vi "Test Classes.vi"() -> ()   [LabVIEW 2009]
uses:
  LV-BME Interface/ChnlSettings.ctl
  LV-BME Interface/BME_DG_TriggerSettings.ctl
  LV-BME Interface/ClockSource.ctl
  DG Classes/BME_DG_System/BME_DG_System.lvclass
  DG Classes/BME_DG_Base/BME_DG_Base.lvclass
  DG Classes/BME_DG_Chnl/BME_DG_Chnl.lvclass
panel:
  in  "SetDelay":bool=TRUE
  in  "UpdateChnl 2":bool=TRUE
  in  "ChnlParameter":T2 {"ChnParam2write"."Delay (µs)" min=0.0 max=100000000.0 format="%.5f"}
  out "CountsRemains":i32
  in  "Acknowledge Interrupts":bool=TRUE
  out "TriggerCounters":i32[](array[numeric])
  out "Interrupts":u32[](array[numeric]) format="%b"
  in  "ClockSource Master":T3=1 items=["Internal Oscillator"=1, "External Trigger"=2, "Trigger & Oscillator"=3, "MasterSlave Bus"=4]
  in  "Trigger Settings Slaves":T4={"InputTerminated?"=FALSE, "InternalClockPeriode(µs)"=1000000.0, "TriggerLevel"=1.25, "PresetValue"=0, "DivideBy"=1, "Clock Source"=1, "Gate Divider"=1, "PositiveGate?"=TRUE, "InternalTrigger?"=FALSE, "InternalArm?"=FALSE, "SWTrigger?"=FALSE, "RisingEdge?"=FALSE, "StopOnPreset?"=FALSE, "ResetWhenDone?"=TRUE, "TriggerEnabled?"=TRUE} {"Gate Divider" min=1 max=1000000; "Clock Source" items=["Internal Oscillator"=1, "External Trigger"=2, "Trigger & Oscillator"=3]}
  in  "Trigger Settings Master":T4={"InputTerminated?"=FALSE, "InternalClockPeriode(µs)"=1000000.0, "TriggerLevel"=1.25, "PresetValue"=0, "DivideBy"=1, "Clock Source"=1, "Gate Divider"=1, "PositiveGate?"=TRUE, "InternalTrigger?"=TRUE, "InternalArm?"=FALSE, "SWTrigger?"=FALSE, "RisingEdge?"=FALSE, "StopOnPreset?"=FALSE, "ResetWhenDone?"=TRUE, "TriggerEnabled?"=TRUE} {"Gate Divider" min=1 max=1000000; "Clock Source" items=["Internal Oscillator"=1, "External Trigger"=2, "Trigger & Oscillator"=3]}
  out "RemainingTriggers":T5(array[cluster])=[[{"Time Stamp"=timestamp(3416308194.6875 s since 1904-01-01), "Numeric"=-64}, {"Time Stamp"=timestamp(3416308194.6875 s since 1904-01-01), "Numeric"=4}, {"Time Stamp"=timestamp(3416308194.6875 s since 1904-01-01), "Numeric"=-64}, {"Time Stamp"=timestamp(3416308194.6875 s since 1904-01-01), "Numeric"=-64}], [{"Time Stamp"=timestamp(3416308194.6875 s since 1904-01-01), "Numeric"=-64}, {"Time Stamp"=timestamp(3416308194.6875 s since 1904-01-01), "Numeric"=-64}, {"Time Stamp"=timestamp(3416308194.6875 s since 1904-01-01), "Numeric"=-64}, {"Time Stamp"=timestamp(3416308194.6875 s since 1904-01-01), "Numeric"=-64}], [{"Time Stamp"=timestamp(3416308194.6875 s since 1904-01-01), "Numeric"=-64}, {"Time Stamp"=timestamp(3416308194.6875 s since 1904-01-01), "Numeric"=-64}, {"Time Stamp"=timestamp(3416308194.6875 s since 1904-01-01), "Numeric"=-64}, {"Time Stamp"=timestamp(3416308194.6875 s since 1904-01-01), "Numeric"=-64}]] {"Time Stamp" format="%<%I:%M:%S%3u %p>T"}
  in  "stop 2":bool=TRUE
  in  "ReadStatus":bool=TRUE
  in  "Activate":bool
  in  "UpdateChnl":bool=TRUE
  in  "TriggerModulo":u32=4
  out "Modulo Settings":u32[](array[numeric])
  out "Chnls":T1[](array[typedef])=[{" Delay (µs)"=0.0, "On? (false)"=TRUE, "PositiveVoltage?(true)"=TRUE, "50OhmTerminated? "=TRUE, "25OhmOutput?"=FALSE}, {" Delay (µs)"=0.0, "On? (false)"=TRUE, "PositiveVoltage?(true)"=TRUE, "50OhmTerminated? "=TRUE, "25OhmOutput?"=FALSE}, {" Delay (µs)"=0.0, "On? (false)"=TRUE, "PositiveVoltage?(true)"=TRUE, "50OhmTerminated? "=TRUE, "25OhmOutput?"=FALSE}] {"Delay (µs)" min=0.0 max=100000000.0 format="%.5f"}
  in  "Trigger Base":T4={"InputTerminated?"=FALSE, "InternalClockPeriode(µs)"=1000000.0, "TriggerLevel"=1.25, "PresetValue"=0, "DivideBy"=1, "Clock Source"=1, "Gate Divider"=1, "PositiveGate?"=TRUE, "InternalTrigger?"=FALSE, "InternalArm?"=FALSE, "SWTrigger?"=FALSE, "RisingEdge?"=FALSE, "StopOnPreset?"=FALSE, "ResetWhenDone?"=TRUE, "TriggerEnabled?"=TRUE} {"Gate Divider" min=1 max=1000000; "Clock Source" items=["Internal Oscillator"=1, "External Trigger"=2, "Trigger & Oscillator"=3]}
  in  "Selected Chnl":u16(ring) items=["Slave 1_ChnlT0", "Slave 1_ChnlA", "Slave 1_ChnlB"]
  in  "Selected Card":u16(ring)=1 items=["Master", "Slave 1", "Slave 2", "Slave 3"]
  in  "STOP":bool=TRUE
  in  "ChnParam2write":T1={" Delay (µs)"=0.0, "On? (false)"=TRUE, "PositiveVoltage?(true)"=TRUE, "50OhmTerminated? "=TRUE, "25OhmOutput?"=FALSE} {"Delay (µs)" min=0.0 max=100000000.0 format="%.5f"}
  # "INIT Values"
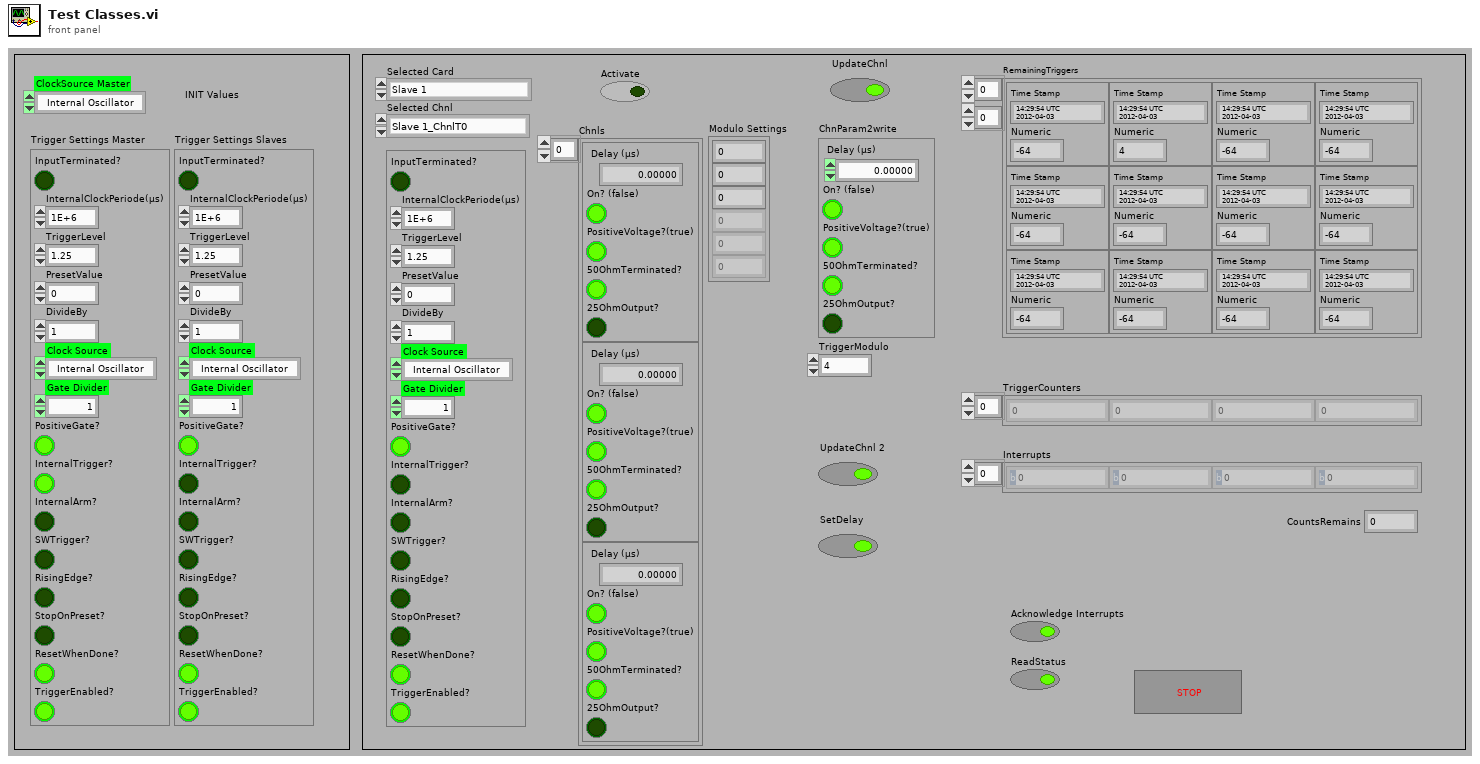
[diagram p1: front panel]
types:
  T1 = typedef "ChnlSettings.ctl" = cluster{" Delay (µs)":dbl, "On? (false)":bool, "PositiveVoltage?(true)":bool, "50OhmTerminated? ":bool, "25OhmOutput?":bool}
  T2 = cluster{"ChnlName":string, "ChnParam2write":T1, "TriggerModulo":u32}
  T3 = typedef "ClockSource.ctl" = i32
  T4 = typedef "BME_DG_TriggerSettings.ctl" = cluster{"InputTerminated?":bool, "InternalClockPeriode(µs)":dbl, "TriggerLevel":dbl, "PresetValue":i32, "DivideBy":i32, "Clock Source":u32, "Gate Divider":i32, "PositiveGate?":bool, "InternalTrigger?":bool, "InternalArm?":bool, "SWTrigger?":bool, "RisingEdge?":bool, "StopOnPreset?":bool, "ResetWhenDone?":bool, "TriggerEnabled?":bool}
  T5 = cluster{"Time Stamp":timestamp, "Numeric":i32}[][]
  T6 = enum8{"Enabled", "Disabled", "Disabled and Grayed Out"}
  T7 = cluster{"ChnlName":string, "ChnParam2write":T1, "TriggerModulo":u32}[]
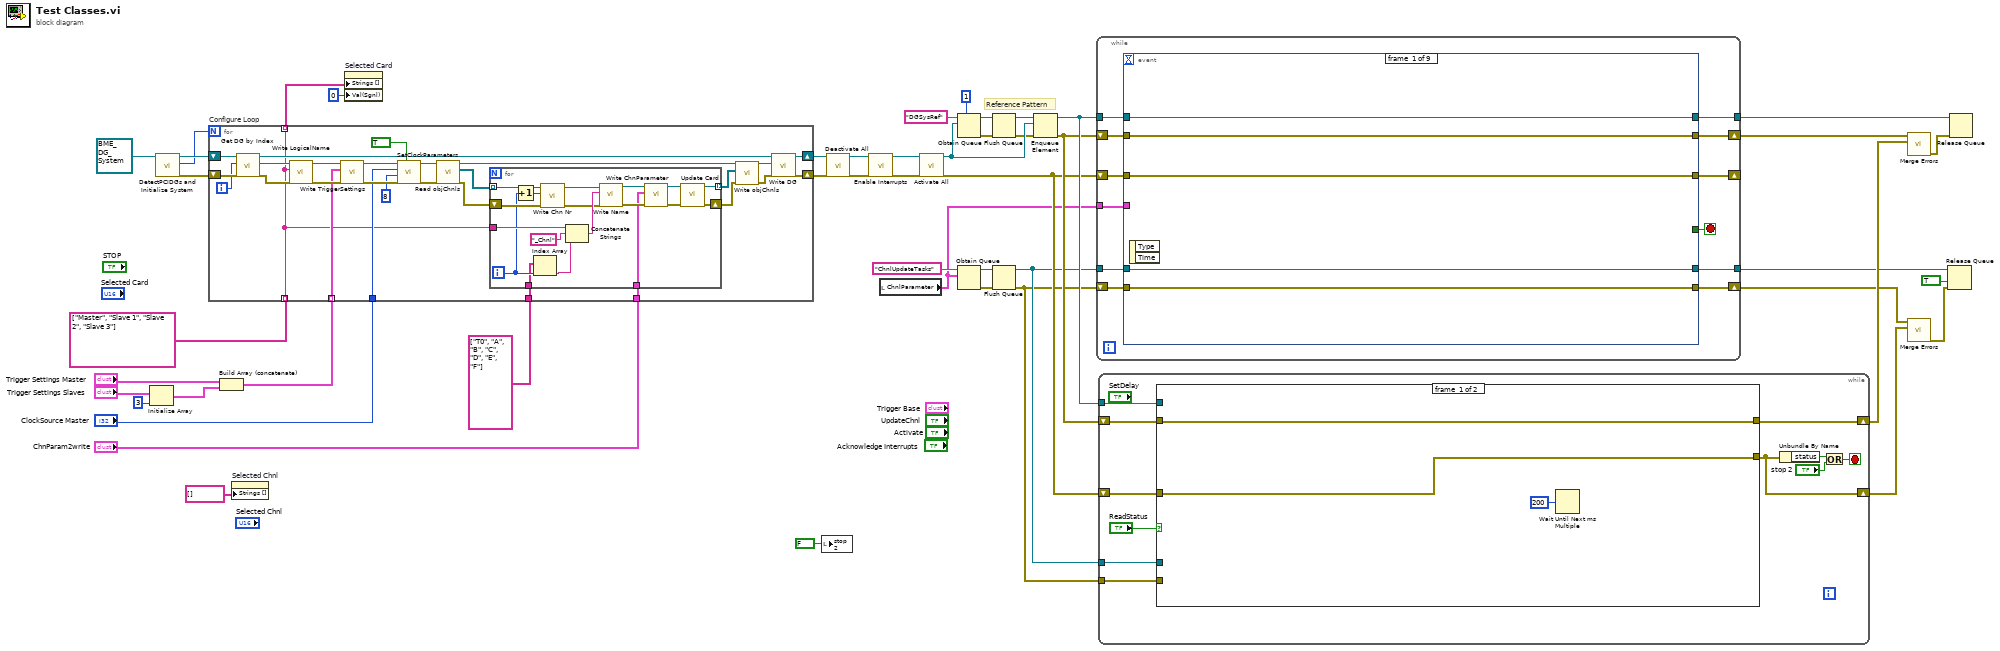
[diagram p0: block diagram]
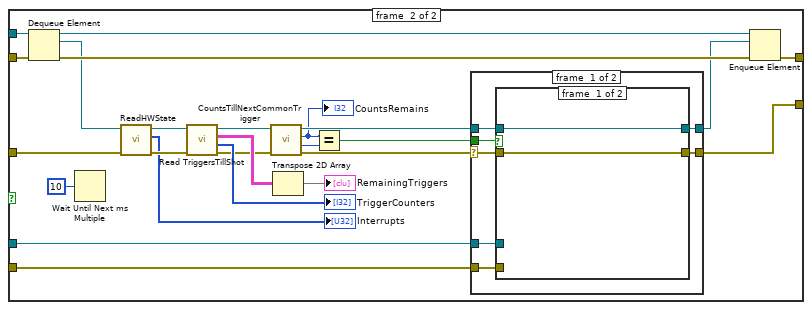
[diagram p2: hidden frame]
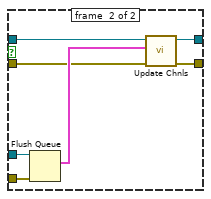
[diagram p3: hidden frame]
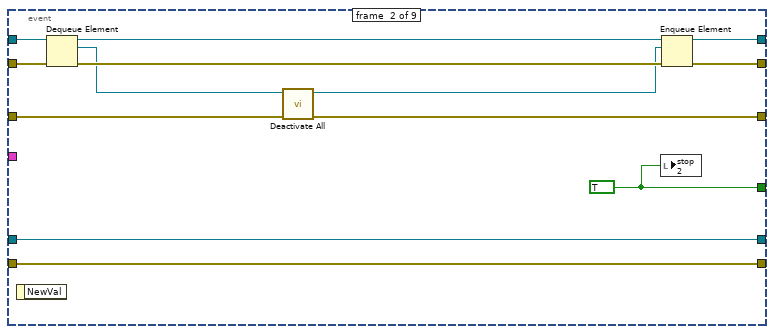
[diagram p5: hidden frame]
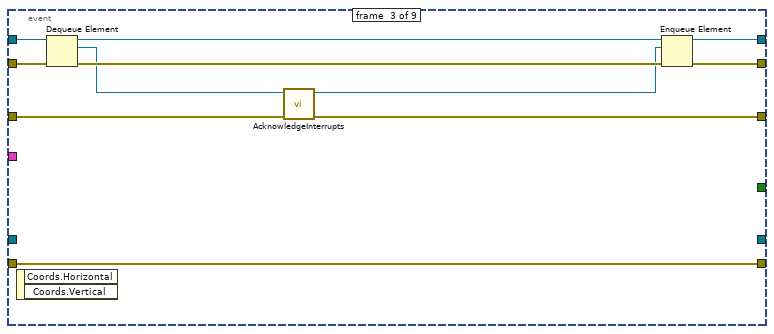
[diagram p6: hidden frame]
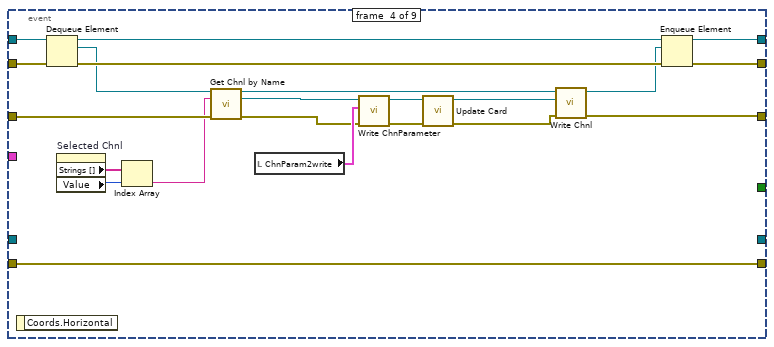
[diagram p7: hidden frame]
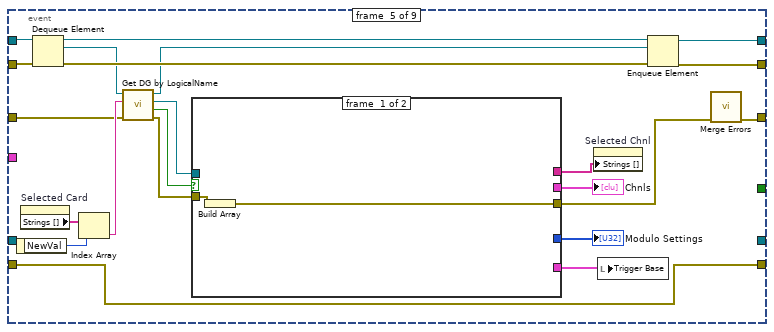
[diagram p8: hidden frame]
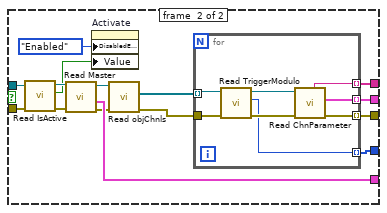
[diagram p9: hidden frame]
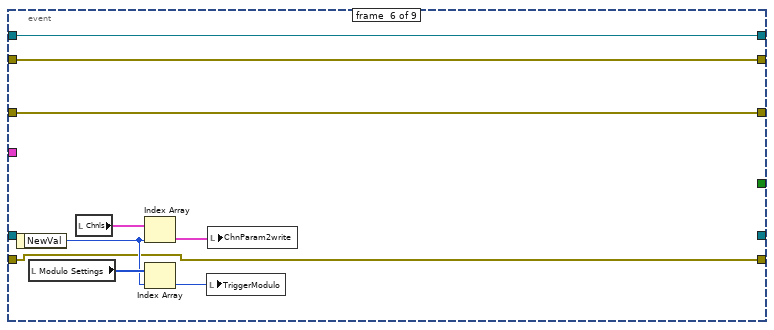
[diagram p10: hidden frame]
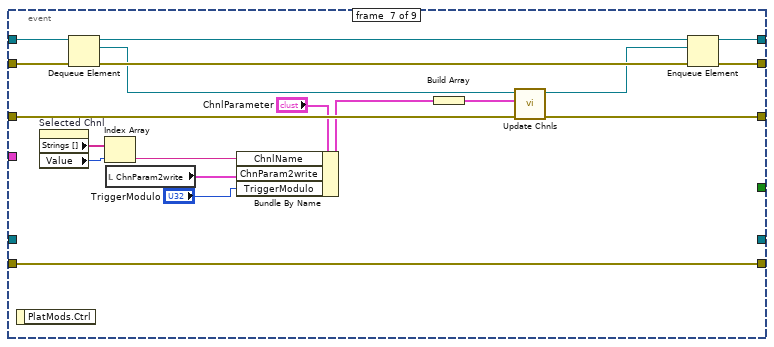
[diagram p11: hidden frame]
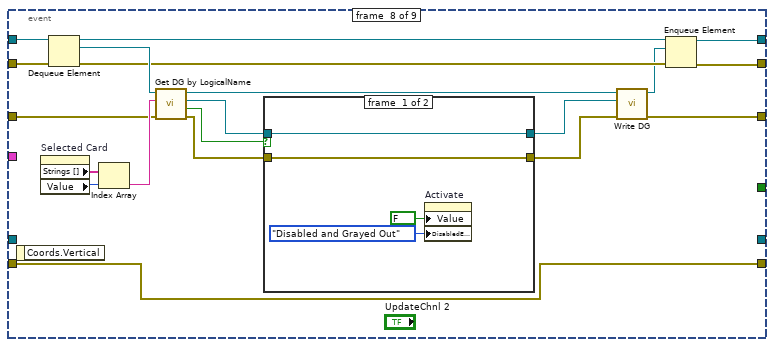
[diagram p12: hidden frame]
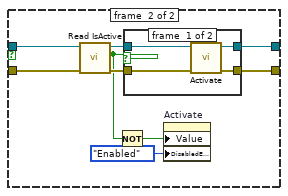
[diagram p13: hidden frame]
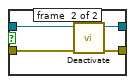
[diagram p14: hidden frame]
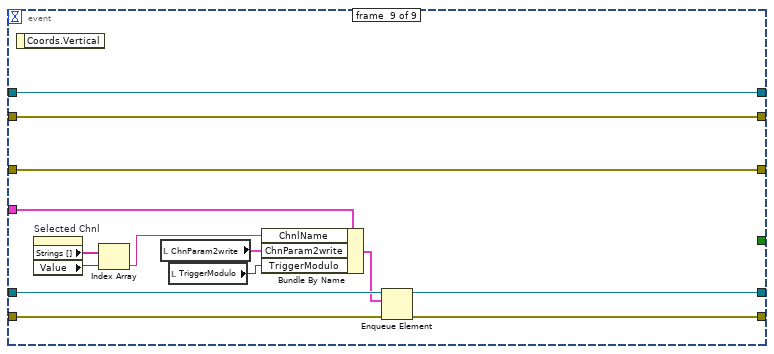
[diagram p15: hidden frame]
diagram:
  # "Reference Pattern"
  n1 = Initialize Array("Trigger Settings Slaves", 3 ("dimension size")) -> (w18:T4[])
  n2 = call "DetectPCIDGs and Initialize System.vi"("BME_DG_System in"=refnum<class "BME_DG_System.lvclass"> refnum ("BME_DG_System.lvclass")) -> ("error out"=w46:errorcluster, "NumberOfCards"=w45:i32, "BME_DG_System out"=w47:refnum<class "BME_DG_System.lvclass">)  [unwired: 8 in]
  n3 = Build Array (concatenate)("Trigger Settings Master", w18) -> (w21:T4[])
  n4 = for "Configure Loop" {
    N: w45 -> [_]
    shift-right: [w62] -> w39
    shift-left: w47 -> [w76]
    tunnel: string[] ["Master", "Slave 1", "Slave 2", "Slave 3"] -> [w49] mode=indexing
    tunnel: w21 -> [w67] mode=indexing
    tunnel: "ClockSource Master" -> [w64]
    shift-right: [w61] -> w38
    shift-left: w46 -> [w75]
    tunnel: "ChnParam2write" -> [w56]
    tunnel: string[] ["T0", "A", "B", "C", "D", "E", "F"] -> [w50]
    tunnel: [w49] -> w41 mode=indexing
    i -> [w74]
    n5 = call "Get DG by Index.vi"("error in (no error)"=w75, "index"=w74, "BME_DG_System in"=w76) -> ("error out"=w70:errorcluster, "BME_DG_Base.lvclass"=w73:refnum<class "BME_DG_Base.lvclass">, "BME_DG_System out"=w63:refnum<class "BME_DG_System.lvclass">)  [unwired: 6 in]
    n6 = call "Write LogicalName.vi"("error in (no error)"=w70, "LogicalName"=w49, "BME_DG_Base in"=w73) -> ("error out"=w69:errorcluster, "BME_DG_Base out"=w72:refnum<class "BME_DG_Base.lvclass">)  [unwired: 7 in]
    n7 = call-dynamic "Write TriggerSettings.vi"("error in (no error)"=w69, "Trigger Settings"=w67, "BME_DG_Base in"=w72) -> ("error out"=w68:errorcluster, "BME_DG_Base out"=w71:refnum<class "BME_DG_Base.lvclass">)  [unwired: 7 in]
    n8 = call-dynamic "SetClockParameters.vi"("ClockEnable"=TRUE, "error in (no error)"=w68, "DivideBy"=u32 8, "ClockSource"=w64, "BME_DG_Base in"=w71) -> ("error out"=w59:errorcluster, "BME_DG_Base out"=w60:refnum<class "BME_DG_Base.lvclass">)  [unwired: 5 in]
    n9 = call-dynamic "Read objChnls.vi"("error in (no error)"=w59, "BME_DG_Base in"=w60) -> ("error out"=w57:errorcluster, "objChnls"=w58:refnum<class "BME_DG_Chnl.lvclass">[], "BME_DG_Base out"=w54:refnum<class "BME_DG_Base.lvclass">)  [unwired: 6 in, 1 out]
    n10 = for {
      tunnel: w58 -> [w88] mode=indexing
      shift-right: [w77] -> w52
      shift-left: w57 -> [w86]
      tunnel: w49 -> [w93]
      tunnel: w56 -> [w89]
      tunnel: [w79] -> w55 mode=indexing
      tunnel: w50 -> [w82]
      i -> [w83]
      n11 = Increment(x=w83) -> (x+1=w84:i32)
      n12 = Index Array(array=w82, index=w83) -> (element=w81:string)
      n13 = call-dynamic "Write Chn Nr.vi"("error in (no error)"=w86, "Chn Nr"=w84, "BME_DG_Chnl in"=w88) -> ("error out"=w85:errorcluster, "BME_DG_Chnl out"=w87:refnum<class "BME_DG_Chnl.lvclass">)  [unwired: 7 in]
      n14 = Concatenate Strings(w93, "_Chnl" ("string"), w81) -> (w91:string)
      n15 = call-dynamic "Write Name.vi"("error in (no error)"=w85, "Name"=w91, "BME_DG_Chnl in"=w87) -> ("error out"=w90:errorcluster, "BME_DG_Chnl out"=w94:refnum<class "BME_DG_Chnl.lvclass">)  [unwired: 7 in]
      n16 = call-dynamic "Write ChnParameter.vi"("error in (no error)"=w90, "ChnParemater"=w89, "BME_DG_Chnl in"=w94) -> ("error out"=w78:errorcluster, "BME_DG_Chnl out"=w80:refnum<class "BME_DG_Chnl.lvclass">)  [unwired: 7 in]
      n17 = call-dynamic "Update Card.vi"("error in (no error)"=w78, "BME_DG_Chnl in"=w80) -> ("error out"=w77:errorcluster, "BME_DG_Chnl out"=w79:refnum<class "BME_DG_Chnl.lvclass">)  [unwired: 8 in]
    }
    n18 = call-dynamic "Write objChnls.vi"("error in (no error)"=w52, "objChnls"=w55, "BME_DG_Base in"=w54) -> ("error out"=w51:errorcluster, "BME_DG_Base out"=w53:refnum<class "BME_DG_Base.lvclass">)  [unwired: 7 in]
    n19 = call "Write DG.vi"("error in (no error)"=w51, "BME_DG_Base"=w53, "BME_DG_System in"=w63) -> ("error out"=w61:errorcluster, "BME_DG_System out"=w62:refnum<class "BME_DG_System.lvclass">)  [unwired: 7 in]
  }
  n20 = property on="Selected Chnl" class="Ring (strict)"("Strings []"=string[] []) -> ()  [unwired: 2 in, 2 out]
  n21 = property on="Selected Card" class="Ring (strict)"("Strings []"=w41, "Val(Sgnl)"=u16 0 ("Value (Signaling)")) -> ()  [unwired: 2 in, 2 out]
  n22 = local write "stop 2"(FALSE ("stop 2")) -> ()
  n23 = call "Deactivate All.vi"("error in (no error)"=w38, "BME_DG_System in"=w39) -> ("error out"=w12:errorcluster, "BME_DG_System out"=w15:refnum<class "BME_DG_System.lvclass">)  [unwired: 8 in]
  n24 = call "Enable Interrupts.vi"("error in (no error)"=w12, "BME_DG_System in"=w15) -> ("error out"=w13:errorcluster, "BME_DG_System out"=w14:refnum<class "BME_DG_System.lvclass">)  [unwired: 8 in]
  n25 = local read "ChnlParameter"() -> (w8:T2)
  n26 = call "Activate All.vi"("error in (no error)"=w13, "BME_DG_System in"=w14) -> ("error out"=w28:errorcluster, "BME_DG_System out"=w35:refnum<class "BME_DG_System.lvclass">)  [unwired: 8 in]
  n27 = Obtain Queue(max queue size (-1, unlimited)=1, name (unnamed)="DGSysRef", element data type=w35) -> (queue out=w26:refnum<queue>, error out=w24:errorcluster)  [unwired: 2 in, 1 out]
  n28 = Obtain Queue(name (unnamed)="ChnlUpdateTasks", element data type=w8) -> (queue out=w9:refnum<queue>, error out=w10:errorcluster)  [unwired: 3 in, 1 out]
  n29 = Flush Queue(queue=w26, error in (no error)=w24) -> (queue out=w25:refnum<queue>, error out=w23:errorcluster)  [unwired: 1 out]
  n30 = Flush Queue(queue=w9, error in (no error)=w10) -> (queue out=w5:refnum<queue>, error out=w4:errorcluster)  [unwired: 1 out]
  n31 = Enqueue Element(queue=w25, element=w35, error in (no error)=w23) -> (queue out=w34:refnum<queue>, error out=w33:errorcluster)  [unwired: 1 in, 1 out]
  n32 = while {
    shift-right: [w102] -> _
    shift-left: w28 -> [w104]
    shift-right: [w100] -> w30
    shift-left: w33 -> [w101]
    tunnel: w34 -> [w105]
    tunnel: [w103] -> w32
    tunnel: w5 -> [w99]
    tunnel: w8 -> [w98]
    tunnel: [w96] -> w7
    shift-right: [w95] -> w3
    shift-left: w4 -> [w97]
    stop <- w106 stop-if-true
    n33 = event shown="[3] \"SetDelay\": Mouse Down" {
      selector: _ -> [_ _ _ _ _ _ _ _ _]
      dyn-events: _ -> [_ _ _ _ _ _ _ _ _]
      timeout: _ -> [_ _ _ _ _ _ _ _ _]
      tunnel: [_ w114 _ _ _ _ _ _ _] -> w106
      tunnel: w105 -> [w111 w121 w134 w156 w167 w213 w230 w241 w287]
      tunnel: w104 -> [w110 w124 w126 w147 w176 w212 w222 w249 w286]
      tunnel: [w111 w117 w130 w152 w165 w213 w225 w235 w287] -> w103
      tunnel: [w110 w123 w127 w136 w160 w212 w221 w242 w286] -> w102
      tunnel: w101 -> [w109 w120 w133 w155 w166 w206 w228 w240 w283]
      tunnel: [w109 w118 w131 w153 w164 w206 w226 w234 w283] -> w100
      tunnel: w99 -> [w108 w113 _ _ _ _ _ _ w278]
      tunnel: w98 -> [_ _ _ _ _ _ _ _ w282]
      tunnel: w97 -> [w107 w112 w125 w151 w158 w205 w215 w233 w276]
      tunnel: [w108 w113 _ _ _ _ _ _ w275] -> w96
      tunnel: [w107 w112 w125 w151 w158 w205 w215 w233 w274] -> w95
      event #0 {
        n34 = event-data() -> ()  [unwired: 1 in, 2 out]
      }
      event #1 {
        w114 = TRUE
        n35 = event-data() -> ()  [unwired: 1 in, 1 out]
        n36 = Dequeue Element(queue=w121, error in (no error)=w120) -> (queue out=w122:refnum<queue>, element=w115:refnum<class "BME_DG_System.lvclass">, error out=w119:errorcluster)  [unwired: 1 in, 1 out]
        n37 = call "Deactivate All.vi"("error in (no error)"=w124, "BME_DG_System in"=w115) -> ("error out"=w123:errorcluster, "BME_DG_System out"=w116:refnum<class "BME_DG_System.lvclass">)  [unwired: 8 in]
        n38 = local write "stop 2"(w114) -> ()
        n39 = Enqueue Element(queue=w122, element=w116, error in (no error)=w119) -> (queue out=w117:refnum<queue>, error out=w118:errorcluster)  [unwired: 1 in, 1 out]
      }
      event #2 {
        n40 = event-data() -> ()  [unwired: 1 in, 2 out]
        n41 = Dequeue Element(queue=w134, error in (no error)=w133) -> (queue out=w135:refnum<queue>, element=w129:refnum<class "BME_DG_System.lvclass">, error out=w132:errorcluster)  [unwired: 1 in, 1 out]
        n42 = call "AcknowledgeInterrupts.vi"("error in (no error)"=w126, "BME_DG_System in"=w129) -> ("error out"=w127:errorcluster, "BME_DG_System out"=w128:refnum<class "BME_DG_System.lvclass">)  [unwired: 8 in]
        n43 = Enqueue Element(queue=w135, element=w128, error in (no error)=w132) -> (queue out=w130:refnum<queue>, error out=w131:errorcluster)  [unwired: 1 in, 1 out]
      }
      event #3 {
        n44 = event-data() -> ()  [unwired: 1 in, 1 out]
        n45 = Dequeue Element(queue=w156, error in (no error)=w155) -> (queue out=w157:refnum<queue>, element=w148:refnum<class "BME_DG_System.lvclass">, error out=w154:errorcluster)  [unwired: 1 in, 1 out]
        n46 = property on="Selected Chnl" class="Ring (strict)"() -> ("Strings []"=w149:string[], "Value"=w150:u16)  [unwired: 2 in, 2 out]
        n47 = Index Array(array=w149, index=w150) -> (element=w146:string)
        n48 = call "Get Chnl by Name.vi"("BME_DG_System in"=w148, "Chnl Name"=w146, "error in (no error)"=w147) -> ("BME_DG_System out"=w142:refnum<class "BME_DG_System.lvclass">, "BME_DG_Chnl"=w145:refnum<class "BME_DG_Chnl.lvclass">, "error out"=w143:errorcluster)  [unwired: 7 in, 3 out]
        n49 = local read "ChnParam2write"() -> (w144:T1)
        n50 = call-dynamic "Write ChnParameter.vi"("error in (no error)"=w143, "ChnParemater"=w144, "BME_DG_Chnl in"=w145) -> ("error out"=w139:errorcluster, "BME_DG_Chnl out"=w140:refnum<class "BME_DG_Chnl.lvclass">)  [unwired: 7 in]
        n51 = call-dynamic "Update Card.vi"("error in (no error)"=w139, "BME_DG_Chnl in"=w140) -> ("error out"=w137:errorcluster, "BME_DG_Chnl out"=w138:refnum<class "BME_DG_Chnl.lvclass">)  [unwired: 8 in]
        n52 = call "Write Chnl.vi"("error in (no error)"=w137, "BME_DG_Chnl.lvclass"=w138, "BME_DG_System in"=w142) -> ("error out"=w136:errorcluster, "BME_DG_System out"=w141:refnum<class "BME_DG_System.lvclass">)  [unwired: 7 in]
        n53 = Enqueue Element(queue=w157, element=w141, error in (no error)=w154) -> (queue out=w152:refnum<queue>, error out=w153:errorcluster)  [unwired: 1 in, 1 out]
      }
      event #4 {
        n54 = event-data() -> ("NewVal"=w178:u16)  [unwired: 1 in]
        n55 = property on="Selected Card" class="Ring (strict)"() -> ("Strings []"=w179:string[])  [unwired: 2 in, 2 out]
        n56 = Dequeue Element(queue=w167, error in (no error)=w166) -> (queue out=w168:refnum<queue>, element=w163:refnum<class "BME_DG_System.lvclass">, error out=w169:errorcluster)  [unwired: 1 in, 1 out]
        n57 = Index Array(array=w179, index=w178) -> (element=w177:string)
        n58 = call "Get DG by LogicalName.vi"("error in (no error)"=w176, "LogicalName"=w177, "BME_DG_System in"=w163) -> ("error out"=w161:errorcluster, "found?"=w175:bool, "BME_DG_Base.lvclass"=w174:refnum<class "BME_DG_Base.lvclass">, "BME_DG_System out"=w162:refnum<class "BME_DG_System.lvclass">)  [unwired: 5 in]
        n59 = case shown="True" w175 {
          tunnel: w174 -> [_ w189]
          tunnel: [_ w196] -> w173
          tunnel: [_ w195] -> w171
          tunnel: [_ w194] -> w172
          tunnel: [_ w190] -> w170
          tunnel: w161 -> [w181 w186]
          tunnel: [w180 w184] -> w159
          frame #0 {
            n60 = Build Array(w181) -> (w180:errorcluster[])
          }
          frame #1 {
            n61 = call-dynamic "Read IsActive.vi"("error in (no error)"=w186, "BME_DG_Base in"=w189) -> ("error out"=w187:errorcluster, "Active?"=w182:bool, "BME_DG_Base out"=w188:refnum<class "BME_DG_Base.lvclass">)  [unwired: 7 in]
            n62 = call-dynamic "Read Master.vi"("error in (no error)"=w187, "BME_DG_Base in"=w188) -> ("error out"=w191:errorcluster, "TriggerSettings"=w194:T4, "BME_DG_Base out"=w192:refnum<class "BME_DG_Base.lvclass">)  [unwired: 6 in, 1 out]
            n63 = property on="Activate" class="Bool (strict)"("DisabledEnum"=T6."Enabled" ("Disabled"), "Value"=w182) -> ()  [unwired: 2 in, 2 out]
            n64 = call-dynamic "Read objChnls.vi"("error in (no error)"=w191, "BME_DG_Base in"=w192) -> ("error out"=w185:errorcluster, "objChnls"=w193:refnum<class "BME_DG_Chnl.lvclass">[])  [unwired: 6 in, 2 out]
            n65 = for {
              tunnel: w193 -> [w202] mode=indexing
              tunnel: [w204] -> w196 mode=indexing
              tunnel: [w203] -> w195 mode=indexing
              tunnel: [w197] -> w190 mode=indexing
              tunnel: w185 -> [w200]
              tunnel: [w198] -> w184 mode=indexing
              n66 = call-dynamic "Read TriggerModulo.vi"("error in (no error)"=w200, "BME_DG_Chnl in"=w202) -> ("error out"=w199:errorcluster, "TriggerModulo"=w197:i32, "BME_DG_Chnl out"=w201:refnum<class "BME_DG_Chnl.lvclass">)  [unwired: 7 in]
              n67 = call-dynamic "Read ChnParameter.vi"("error in (no error)"=w199, "BME_DG_Chnl in"=w201) -> ("error out"=w198:errorcluster, "ChnParemater"=w203:T1, "Name"=w204:string)  [unwired: 4 in, 3 out]
            }
          }
        }
        "Chnls" <- w171
        "Modulo Settings" <- w170
        n68 = property on="Selected Chnl" class="Ring (strict)"("Strings []"=w173) -> ()  [unwired: 2 in, 2 out]
        n69 = local write "Trigger Base"(w172) -> ()
        n70 = Enqueue Element(queue=w168, element=w162, error in (no error)=w169) -> (queue out=w165:refnum<queue>, error out=w164:errorcluster)  [unwired: 1 in, 1 out]
        n71 = call <vilib>:"Merge Errors.vi"("error array in"=w159) -> ("error out"=w160:errorcluster)  [unwired: 6 in]
      }
      event #5 {
        n72 = event-data() -> ("NewVal"=w209:u16)  [unwired: 1 in]
        n73 = local read "Modulo Settings"() -> (w210:u32[])
        n74 = local read "Chnls"() -> (w211:T1[])
        n75 = Index Array(array=w211, index=w209) -> (element=w208:T1)
        n76 = Index Array(array=w210, index=w209) -> (element=w207:u32)
        n77 = local write "TriggerModulo"(w207) -> ()
        n78 = local write "ChnParam2write"(w208) -> ()
      }
      event #6 {
        n79 = event-data() -> ()  [unwired: 1 in, 1 out]
        n80 = property on="Selected Chnl" class="Ring (strict)"() -> ("Strings []"=w232:string[], "Value"=w231:u16)  [unwired: 2 in, 2 out]
        n81 = Dequeue Element(queue=w230, error in (no error)=w228) -> (queue out=w229:refnum<queue>, element=w224:refnum<class "BME_DG_System.lvclass">, error out=w227:errorcluster)  [unwired: 1 in, 1 out]
        n82 = Index Array(array=w232, index=w231) -> (element=w218:string)
        n83 = local read "ChnParam2write"() -> (w217:T1)
        n84 = Bundle By Name(cluster="ChnlParameter", "ChnlName"=w218, "ChnParam2write"=w217, "TriggerModulo"="TriggerModulo") -> (w219:T2)
        n85 = Build Array(w219) -> (w214:T7)
        n86 = call "Update Chnls.vi"("error in (no error)"=w222, "ChnlSettings"=w214, "BME_DG_System in"=w224) -> ("error out"=w221:errorcluster, "BME_DG_System out"=w223:refnum<class "BME_DG_System.lvclass">)  [unwired: 7 in]
        n87 = Enqueue Element(queue=w229, element=w223, error in (no error)=w227) -> (queue out=w225:refnum<queue>, error out=w226:errorcluster)  [unwired: 1 in, 1 out]
      }
      event #7 {
        n88 = event-data() -> ()  [unwired: 1 in, 1 out]
        n89 = property on="Selected Card" class="Ring (strict)"() -> ("Strings []"=w252:string[], "Value"=w251:u16)  [unwired: 2 in, 2 out]
        n90 = Dequeue Element(queue=w241, error in (no error)=w240) -> (queue out=w238:refnum<queue>, element=w239:refnum<class "BME_DG_System.lvclass">, error out=w237:errorcluster)  [unwired: 1 in, 1 out]
        n91 = Index Array(array=w252, index=w251) -> (element=w250:string)
        n92 = call "Get DG by LogicalName.vi"("error in (no error)"=w249, "LogicalName"=w250, "BME_DG_System in"=w239) -> ("error out"=w247:errorcluster, "found?"=w243:bool, "BME_DG_Base.lvclass"=w248:refnum<class "BME_DG_Base.lvclass">, "BME_DG_System out"=w244:refnum<class "BME_DG_System.lvclass">)  [unwired: 5 in]
        n93 = case shown="True" w243 {
          tunnel: w248 -> [w256 w263]
          tunnel: w247 -> [w255 w261]
          tunnel: [w255 w265] -> w246
          tunnel: [w256 w264] -> w245
          frame #0 {
            n94 = property on="Activate" class="Bool (strict)"("Value"=FALSE ("Activate"), "DisabledEnum"=T6."Disabled and Grayed Out" ("Disabled")) -> ()  [unwired: 2 in, 2 out]
          }
          frame #1 {
            n95 = call-dynamic "Read IsActive.vi"("error in (no error)"=w261, "BME_DG_Base in"=w263) -> ("error out"=w260:errorcluster, "Active?"=w259:bool, "BME_DG_Base out"=w262:refnum<class "BME_DG_Base.lvclass">)  [unwired: 7 in]
            n96 = Not(x=w259) -> (.not. x?=w257:bool)
            n97 = case shown="True" w259 {
              tunnel: [w269 w271] -> w265
              tunnel: [w268 w272] -> w264
              tunnel: w262 -> [w267 w273]
              tunnel: w260 -> [w266 w270]
              frame #0 {
                n98 = call-dynamic "Activate.vi"("error in (no error)"=w266, "BME_DG_Base in"=w267) -> ("error out"=w269:errorcluster, "BME_DG_Base out"=w268:refnum<class "BME_DG_Base.lvclass">)  [unwired: 8 in]
              }
              frame #1 {
                n99 = call-dynamic "Deactivate.vi"("error in (no error)"=w270, "BME_DG_Base in"=w273) -> ("error out"=w271:errorcluster, "BME_DG_Base out"=w272:refnum<class "BME_DG_Base.lvclass">)  [unwired: 8 in]
              }
            }
            n100 = property on="Activate" class="Bool (strict)"("Value"=w257, "DisabledEnum"=T6."Enabled" ("Disabled")) -> ()  [unwired: 2 in, 2 out]
          }
        }
        n101 = call "Write DG.vi"("error in (no error)"=w246, "BME_DG_Base"=w245, "BME_DG_System in"=w244) -> ("error out"=w242:errorcluster, "BME_DG_System out"=w236:refnum<class "BME_DG_System.lvclass">)  [unwired: 7 in]
        n102 = Enqueue Element(queue=w238, element=w236, error in (no error)=w237) -> (queue out=w235:refnum<queue>, error out=w234:errorcluster)  [unwired: 1 in, 1 out]
      }
      event #8 {
        n103 = event-data() -> ()  [unwired: 1 in, 1 out]
        n104 = property on="Selected Chnl" class="Ring (strict)"() -> ("Strings []"=w284:string[], "Value"=w285:u16)  [unwired: 2 in, 2 out]
        n105 = Index Array(array=w284, index=w285) -> (element=w281:string)
        n106 = local read "ChnParam2write"() -> (w280:T1)
        n107 = local read "TriggerModulo"() -> (w279:u32)
        n108 = Bundle By Name(cluster=w282, "ChnlName"=w281, "ChnParam2write"=w280, "TriggerModulo"=w279) -> (w277:T2)
        n109 = Enqueue Element(queue=w278, element=w277, error in (no error)=w276) -> (queue out=w275:refnum<queue>, error out=w274:errorcluster)  [unwired: 1 in, 1 out]
      }
    }
  }
  n110 = while {
    tunnel: w34 -> [w295]
    shift-right: [w293] -> w29
    shift-left: w33 -> [w294]
    shift-right: [w290] -> w2
    shift-left: w28 -> [w292]
    tunnel: w5 -> [w289]
    tunnel: w4 -> [w288]
    stop <- w297 stop-if-true
    n111 = case shown="True" "ReadStatus" {
      tunnel: w295 -> [_ w324]
      tunnel: w294 -> [w300 w323]
      tunnel: [w300 w322] -> w293
      tunnel: w292 -> [w299 w320]
      tunnel: [w299 w306] -> w290
      tunnel: w289 -> [_ w310]
      tunnel: w288 -> [_ w309]
      frame #0 {
        n112 = Wait Until Next ms Multiple(millisecond multiple=u32 200) -> ()  [unwired: 1 out]
      }
      frame #1 {
        n113 = Dequeue Element(queue=w324, error in (no error)=w323) -> (queue out=w325:refnum<queue>, element=w321:refnum<class "BME_DG_System.lvclass">, error out=w326:errorcluster)  [unwired: 1 in, 1 out]
        n114 = Wait Until Next ms Multiple(millisecond multiple=u32 10) -> ()  [unwired: 1 out]
        n115 = call "ReadHWState.vi"("error in (no error)"=w320, "BME_DG_System in"=w321) -> ("error out"=w319:errorcluster, "Interrupts"=→"Interrupts":u32[], "BME_DG_System out"=w318:refnum<class "BME_DG_System.lvclass">)  [unwired: 7 in]
        n116 = call "Read TriggersTillShot.vi"("error in (no error)"=w319, "BME_DG_System in"=w318) -> ("error out"=w311:errorcluster, "TriggerCounters"=→"TriggerCounters":i32[], "RemainingTriggers"=w317:T5, "BME_DG_System out"=w312:refnum<class "BME_DG_System.lvclass">)  [unwired: 6 in]
        n117 = call "CountsTillNextCommonTrigger.vi"("error in (no error)"=w311, "BME_DG_System in"=w312) -> ("error out"=w308:errorcluster, "LeastCommonMult"=w303:i32, "CountsRemains"=w304:i32, "BME_DG_System out"=w307:refnum<class "BME_DG_System.lvclass">)  [unwired: 6 in]
        "CountsRemains" <- w304
        n118 = Transpose 2D Array(2D array=w317) -> (transposed array=→"RemainingTriggers":T5)
        n119 = Equal?(x=w304, y=w303) -> (x = y?=w302:bool)
        n120 = case shown="No Error" w308 {
          selector: w308 -> [w330 w343]
          tunnel: w310 -> [w333 _]
          tunnel: w309 -> [w332 _]
          tunnel: w307 -> [w331 w344]
          tunnel: [w329 w343] -> w306
          tunnel: [w328 w344] -> w305
          tunnel: w302 -> [w327 _]
          frame #0 {
            n121 = case shown="True" w327 {
              tunnel: w333 -> [_ w342]
              tunnel: w332 -> [_ w341]
              tunnel: w331 -> [w335 w340]
              tunnel: w330 -> [w334 w338]
              tunnel: [w334 w337] -> w329
              tunnel: [w335 w336] -> w328
              frame #0 {
              }
              frame #1 {
                n122 = Flush Queue(queue=w342, error in (no error)=w341) -> (remaining elements=w339:T7)  [unwired: 2 out]
                n123 = call "Update Chnls.vi"("error in (no error)"=w338, "ChnlSettings"=w339, "BME_DG_System in"=w340) -> ("error out"=w337:errorcluster, "BME_DG_System out"=w336:refnum<class "BME_DG_System.lvclass">)  [unwired: 7 in]
              }
            }
          }
          frame #1 {
          }
        }
        n124 = Enqueue Element(queue=w325, element=w305, error in (no error)=w326) -> (error out=w322:errorcluster)  [unwired: 1 in, 2 out]
      }
    }
    n125 = Unbundle By Name(w290) -> ("status"=w296:bool)
    n126 = Or(x=w296, y="stop 2") -> (x .or. y?=w297:bool)
  }
  n127 = call <vilib>:"Merge Errors.vi"("error in 2 (no error)"=w29, "error in 1 (no error)"=w30) -> ("error out"=w31:errorcluster)  [unwired: 5 in]
  n128 = call <vilib>:"Merge Errors.vi"("error in 2 (no error)"=w2, "error in 1 (no error)"=w3) -> ("error out"=w1:errorcluster)  [unwired: 5 in]
  n129 = Release Queue(queue=w7, force destroy? (F)=TRUE, error in (no error)=w1) -> ()  [unwired: 3 out]
  n130 = Release Queue(queue=w32, error in (no error)=w31) -> ()  [unwired: 1 in, 3 out]
